vi "Post-Init.vi"(8 "error in (no error)":errorcluster, 11 "Instrument Driver in":refnum<class "Instrument Driver.lvclass">) -> (0 "error out":errorcluster, 2 "Init Result":refnum<class "Acquired Result.lvclass">, 3 "Instrument Driver out":refnum<class "Instrument Driver.lvclass">)   [LabVIEW 2016, in "Instrument Driver.lvclass"]
uses:
  Instrument Driver.lvclass
  Results/Acquired Result/Acquired Result.lvclass
  Results/Start Stream Result/Start Stream Result.lvclass
  C:/Github/NHMFL_Core/Libraries/Instruments/Results/Acquired Result/Acquired Result.lvclass
  Instrument Driver.lvclass/Instrument Driver.ctl
  Results/Acquired Result/Acquired Result.lvclass/Acquired Result.ctl
  Results/Start Stream Result/Start Stream Result.lvclass/Start Stream Result.ctl
  Read Group name.vi
  Read Channel names.vi
  Read Timing group name.vi
  Read Cycle period.vi
  Results/Acquired Result/Write Group.vi
  Results/Acquired Result/Write Channels.vi
  Results/Acquired Result/Write Time group.vi
  Results/Start Stream Result/Write dt.vi
  Results/Start Stream Result/Write Configuration.vi
  Read User configuration.vi
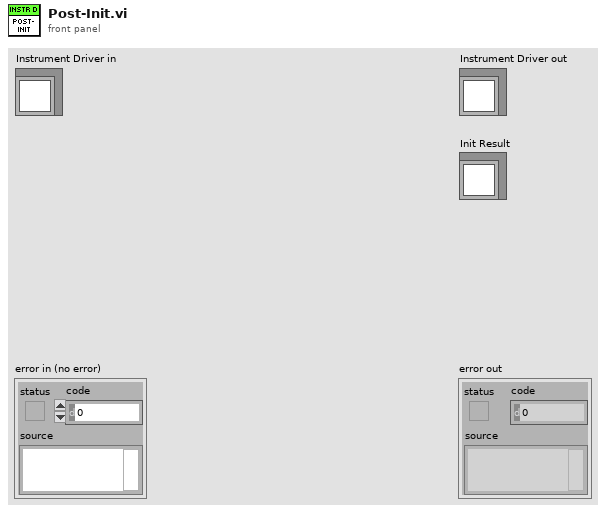
[diagram p1: front panel]
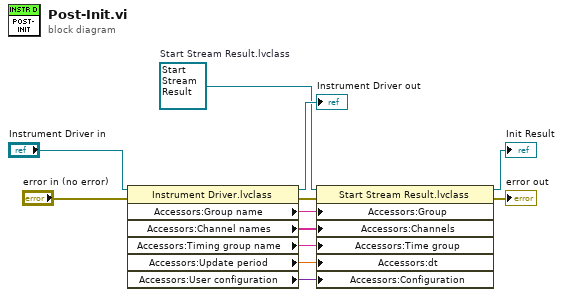
[diagram p0: block diagram]
diagram:
  w3 = refnum<class "Start Stream Result.lvclass"> refnum  # Start Stream Result.lvclass
  n1 = property class="Instrument Driver.lvclass"(reference="Instrument Driver in", error in="error in (no error)") -> (reference out=→"Instrument Driver out":refnum<class "Instrument Driver.lvclass">, error out=w8:errorcluster, "Accessors:Group name"=w9:string, "Accessors:Channel names"=w5:string[], "Accessors:Timing group name"=w4:string, "Accessors:Update period"=w2:dbl, "Accessors:User configuration"=w1:variant)
  n2 = property class="Start Stream Result.lvclass"(reference=w3, error in=w8, "Accessors:Group"=w9, "Accessors:Channels"=w5, "Accessors:Time group"=w4, "Accessors:dt"=w2, "Accessors:Configuration"=w1) -> (reference out=→"Init Result":refnum<class "Start Stream Result.lvclass">, error out=→"error out":errorcluster)
